vi "Sort.vi"() -> ()   [LabVIEW 2018]
panel:
  out "sorted array":string[](array[string])
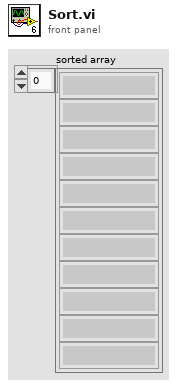
[diagram p1: front panel]
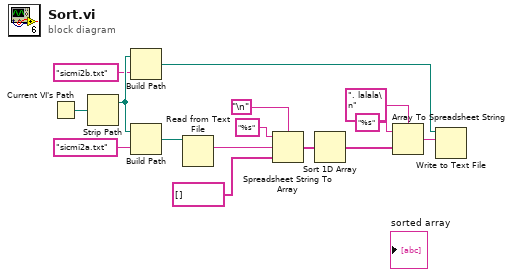
[diagram p0: block diagram]
diagram:
  n1 = Current VI's Path() -> (path=w14:path)
  n2 = Strip Path(path=w14) -> (stripped path=w3:path)  [unwired: 1 out]
  n3 = Build Path(base path=w3, name or relative path="sicmi2b.txt") -> (appended path=w4:path)
  n4 = Build Path(base path=w3, name or relative path="sicmi2a.txt") -> (appended path=w13:path)
  n5 = Read from Text File(file (use dialog)=w13) -> (text=w11:string)  [unwired: 3 in, 3 out]
  n6 = Spreadsheet String To Array(delimiter (Tab)="\n", format string="%s", spreadsheet string=w11, array type (2D Dbl)=string[] []) -> (array=w8:string[])
  n7 = Sort 1D Array(array=w8) -> (sorted array=w6:string[])
  n8 = Array To Spreadsheet String(delimiter (Tab)=". lalala\n", array=w6, 3:"%s" ("format string")) -> (spreadsheet string=w5:string)
  n9 = Write to Text File(file (use dialog)=w4, text=w5) -> ()  [unwired: 2 in, 3 out]
